vi "SeparateInstrumentTest.vi"(8 "test in":string, 9 "Instrument in":string, 10 "Instrument":string, 11 "path in":path) -> (0 "Single Folder?":bool, 1 "Just test":string, 2 "Just Instrument":string, 3 "path out":path, 4 "Instrument -- test out":string)   [LabVIEW 2022 SP3]
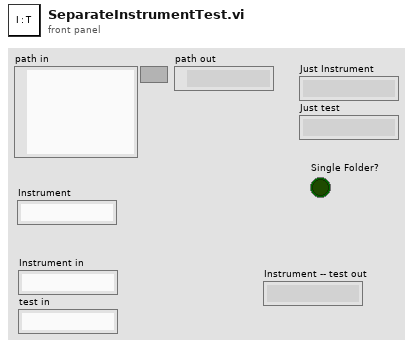
[diagram p1: front panel]
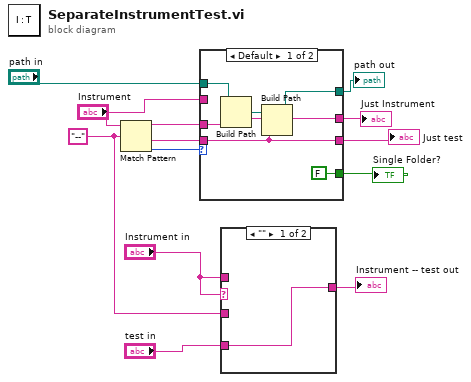
[diagram p0: block diagram]
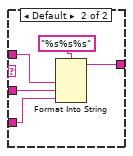
[diagram p2: hidden frame]
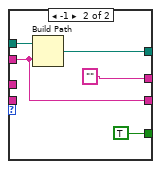
[diagram p3: hidden frame]
diagram:
  w2 = "--" ("regular expression")
  n1 = Match Pattern(string="Instrument", regular expression=w2) -> (before substring=w12:string, after substring=w13:string, offset past match=w8:i32)  [unwired: 1 in, 1 out]
  n2 = case shown="Default" w8 {
    tunnel: "path in" -> [w19 w24]
    tunnel: "Instrument" -> [_ w21]
    tunnel: [w17 w23] -> w11
    tunnel: w12 -> [w16 _]
    tunnel: w13 -> [w15 _]
    tunnel: [w16 "" ("Instrument")] -> w7
    tunnel: [w15 w21] -> w6
    tunnel: [FALSE TRUE] -> w5
    frame Default {
      n3 = Build Path(base path=w19, name or relative path=w16) -> (appended path=w18:path)
      n4 = Build Path(base path=w18, name or relative path=w15) -> (appended path=w17:path)
    }
    frame -1 {
      n5 = Build Path(base path=w24, name or relative path=w21) -> (appended path=w23:path)
    }
  }
  "path out" <- w11
  "Just Instrument" <- w7
  "Just test" <- w6
  "Single Folder?" <- w5
  n6 = case shown="\"\"" "Instrument in" {
    tunnel: "Instrument in" -> [_ w29]
    tunnel: "test in" -> [w25 w28]
    tunnel: [w25 w27] -> w3
    tunnel: w2 -> [_ w26]
    frame "" {
    }
    frame Default {
      n7 = Format Into String(format string="%s%s%s", w29, w26, w28) -> (resulting string=w27:string)  [unwired: 2 in, 1 out]
    }
  }
  "Instrument -- test out" <- w3
